vi "read_serial_check.vi"(7 "checkval":u8=42, 8 "error in (no error)":errorcluster, 10 "byte count":u32, 11 "VISA resource name":refnum<visa-resource-name>) -> (0 "error out":errorcluster, 1 "good":bool, 2 "data":u8[](array[numeric]), 3 "VISA resource out":refnum<visa-resource-name>)   [LabVIEW 2013]
doc: "Use this template to build a VI to use as a subVI."
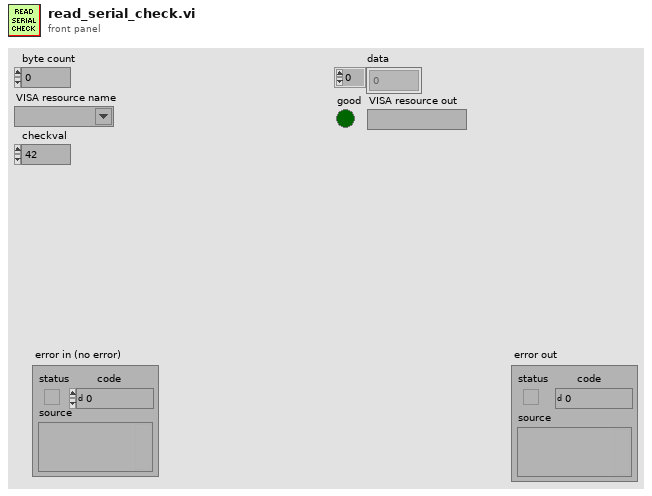
[diagram p1: front panel]
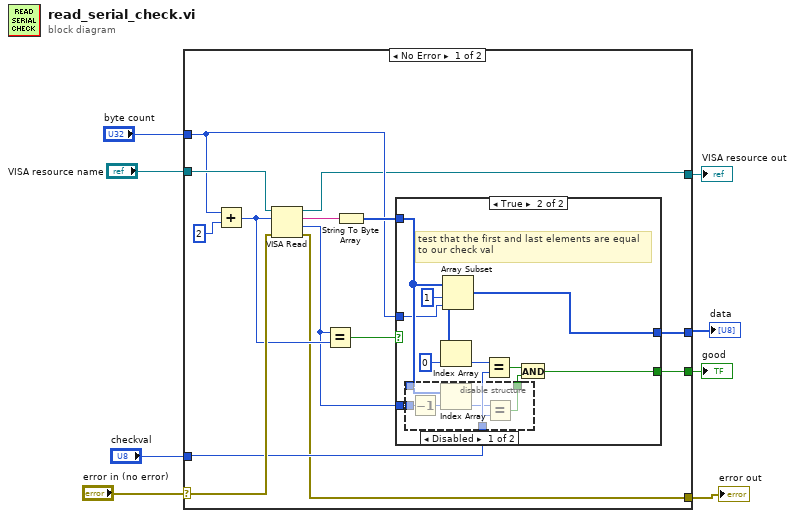
[diagram p0: block diagram]
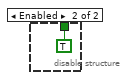
[diagram p3: hidden frame]
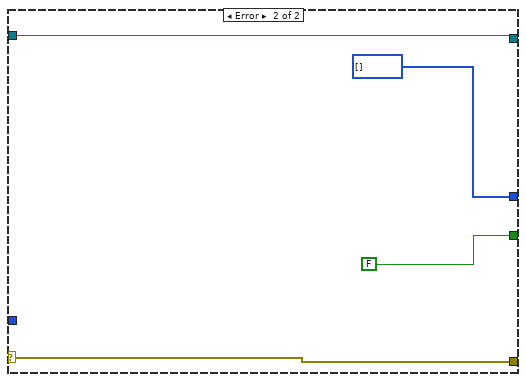
[diagram p4: hidden frame]
diagram:
  n1 = case shown="No Error" "error in (no error)" {
    selector: "error in (no error)" -> [w20 w46]
    tunnel: [w13 w46] -> w7
    tunnel: "byte count" -> [w10 _]
    tunnel: "VISA resource name" -> [w22 w43]
    tunnel: "checkval" -> [w14 _]
    tunnel: [w12 u8[] [] ("unsigned byte array")] -> w3
    tunnel: [w11 FALSE] -> w2
    tunnel: [w9 w43] -> w1
    frame No Error {
      n2 = Add(x=w10, y=u32 2) -> (x+y=w16:u32)
      n3 = VISA Read(VISA resource name=w22, byte count=w16, error in (no error)=w20) -> (VISA resource name out=w9:refnum<visa-resource-name>, read buffer=w19:string, return count=w15:u32, error out=w13:errorcluster)
      n4 = Equal?(x=w15, y=w16) -> (x = y?=w18:bool)
      n5 = String To Byte Array(string=w19) -> (unsigned byte array=w17:u8[])
      n6 = case shown="True" w18 {
        selector: w18 -> [w23 _]
        tunnel: w17 -> [w24 w28]
        tunnel: w15 -> [_ w34]
        tunnel: w14 -> [_ w32]
        tunnel: [w24 w25] -> w12
        tunnel: [w23 w29] -> w11
        tunnel: w10 -> [_ w26]
        frame False {
        }
        frame True {
          # "test that the first and last elements are equal\nto our check val"
          n7 = disable-structure shown="Disabled" {
            disable-tunnel: w34 -> [w40 _]
            disable-tunnel: w32 -> [w38 _]
            disable-tunnel: [w36 TRUE] -> w30
            disable-tunnel: w28 -> [w37 _]
            frame Disabled {
              n8 = Decrement(x=w40) -> (x-1=w41:u32)
              n9 = Index Array(array=w37, index=w41) -> (element=w39:u8)
              n10 = Equal?(x=w39, y=w38) -> (x = y?=w36:bool)
            }
            frame Enabled {
            }
          }
          n11 = Index Array(array=w28, index=0) -> (element=w33:u8)
          n12 = Array Subset(array=w28, index=1, length=w26) -> (w25:u8[])
          n13 = Equal?(x=w33, y=w32) -> (x = y?=w31:bool)
          n14 = And(x=w31, y=w30) -> (x .and. y?=w29:bool)
        }
      }
    }
    frame Error {
    }
  }
  "error out" <- w7
  "data" <- w3
  "good" <- w2
  "VISA resource out" <- w1
